vi "UHR-Fleezers Control (host) - 11.0.vi"() -> ()   [LabVIEW 2011] (continued)
            n1358 = Multiply(x=3276.7, y=w1898) -> (x*y=w1899:cluster{"Set 1":dbl, "Set 2":dbl})
            n1359 = To Word Integer(number=w1899) -> (16bit integer=w1911:cluster{"Set 1":i16, "Set 2":i16})
          }
        }
        n1360 = Unbundle By Name(w1883) -> ("Set 1"=w1882:i16, "Set 2"=w1881:i16)
        n1361 = xnode "Read/Write Control"("FPGA VI Reference In"=w1879, "error in"=w1878, "FB Setpoint Set 1"=w1882, "FB Setpoint Set 2"=w1881) -> ("error out"=w1877:errorcluster)  [unwired: 1 out]
      }
      event "Invert GI": Value Change {
        n1362 = event-data() -> ()  [unwired: 7 out]
        n1363 = xnode "Read/Write Control"("FPGA VI Reference In"=w1916, "error in"=w1914, "Invert GI"="Invert GI", "Invert GI 2"="Invert GI") -> ("error out"=w1915:errorcluster)  [unwired: 1 out]
      }
      event "Green FB Setpoint (mV)", "Green FB Gains", "Green FB On/Off", "Current When FB OFF (%)", "Green int current ON count adj": Value Change {
        n1364 = event-data() -> ()  [unwired: 7 out]
        n1365 = local read "Green FB Setpoint (mV)"() -> (w1923:dbl)
        n1366 = local read "Current When FB OFF (%)"() -> (w1926:dbl)
        n1367 = Multiply(x=w1923, y=3.2767) -> (x*y=w1922:dbl)
        n1368 = Multiply(x=w1926, y=655.35) -> (x*y=w1927:dbl)
        n1369 = To Unsigned Word Integer(number=w1927) -> (unsigned 16bit integer=w1925:u16)
        n1370 = local read "Green int current ON count adj"() -> (w1930:u32)
        n1371 = local read "Green FB Gains"() -> (w1929:T14)
        n1372 = local read "Green Laser ON/Interlacing"() -> (w1920:bool)
        n1373 = local read "Green laser mode"() -> (w1919:enum32{"Laser ON", "Laser OFF", "Interlace"})
        n1374 = local read "Green FB On/Off"() -> (w1931:bool)
        n1375 = Equal?(x=w1919, y=enum32{"Laser ON", "Laser OFF", "Interlace"}."Interlace") -> (x = y?=w1917:bool)
        n1376 = Compound Arithmetic op=AND(w1917, w1931, w1920) -> (w1921:bool)
        n1377 = xnode "Read/Write Control"("FPGA VI Reference In"=w1934, "error in"=w1933, "Green FB Setpoint"=w1922, "Green FB On/Off"=w1921, "Current Out"=w1925, "Green int current ON count adj"=w1930, "Green FB Gains"=w1929) -> ("error out"=w1932:errorcluster)  [unwired: 1 out]
      }
      event "Green laser mode", "Green Laser ON/Interlacing": Value Change {
        n1378 = event-data() -> ()  [unwired: 7 out]
        n1379 = local write "Green Laser ON/OFF"("Green Laser ON/Interlacing") -> ()
        n1380 = case shown="True" "Green Laser ON/Interlacing" {
          tunnel: "Green laser mode" -> [_ w1948]
          tunnel: [enum32{"Laser ON", "Laser OFF", "Interlace"}."Laser OFF" ("Green laser mode") w1948] -> w1937
          tunnel: [FALSE w1944] -> w1936
          frame False {
          }
          frame True {
            n1381 = local read "Green FB On/Off"() -> (w1945:bool)
            n1382 = Equal?(x=w1948, y=enum32{"Laser ON", "Laser OFF", "Interlace"}."Interlace") -> (x = y?=w1946:bool)
            n1383 = And(x=w1946, y=w1945) -> (x .and. y?=w1944:bool)
          }
        }
        n1384 = xnode "Read/Write Control"("FPGA VI Reference In"=w1941, "error in"=w1939, "Operating Mode"=w1937, "Operating Mode 2"=w1937, "Green FB On/Off"=w1936) -> ("error out"=w1940:errorcluster)  [unwired: 1 out]
      }
      event "Green Laser ON/OFF": Value Change {
        n1385 = event-data() -> ()  [unwired: 7 out]
        n1386 = property on="Green Laser ON/Interlacing" class="Bool (strict)"("Val(Sgnl)"="Green Laser ON/OFF") -> ()  [unwired: 2 in, 2 out]
      }
      event "Test ttrig": Value Change {
        n1387 = event-data() -> ()  [unwired: 7 out]
        n1388 = xnode "Read/Write Control"("FPGA VI Reference In"=w1953, "error in"=w1952, "TTrig?"=TRUE) -> ("error out"=w1951:errorcluster)  [unwired: 1 out]
      }
      event "Neg. TTrig FPGA": Value Change {
        n1389 = event-data() -> ()  [unwired: 7 out]
        n1390 = xnode "Read/Write Control"("FPGA VI Reference In"=w1957, "error in"=w1956, "TTrig Negate Pos"="Neg. TTrig FPGA") -> ()  [unwired: 2 out]
      }
      event "- phase (APD 1 Gate)", "+ phase (APD 1 Gate)": Value Change {
        n1391 = event-data() -> ()  [unwired: 7 out]
        n1392 = local read "Phase Adj. (APD 1 Gate)"() -> (w1958:i16)
        n1393 = Negate(x=w1958) -> (-x=w1966:i16)
        n1394 = Select(t=w1966, s="- phase (APD 1 Gate)", f=w1958) -> (s? t:f=w1965:i16)
        n1395 = Or(x="- phase (APD 1 Gate)", y="+ phase (APD 1 Gate)") -> (x .or. y?=w1961:bool)
        n1396 = xnode "Read/Write Control"("FPGA VI Reference In"=w1968, "error in"=w1967, "Phase count adjustment (APD 1 Gate)"=w1965) -> ("FPGA VI Reference Out"=w1963:T19, "error out"=w1964:errorcluster)
        n1397 = xnode "Read/Write Control"("FPGA VI Reference In"=w1963, "error in"=w1964, "+ phase (APD 1 Gate)"=w1961) -> ("error out"=w1962:errorcluster)  [unwired: 1 out]
      }
      event "+ phase (APD 2 Gate)", "- phase (APD 2 Gate)": Value Change {
        n1398 = event-data() -> ()  [unwired: 7 out]
        n1399 = local read "Phase Adj. (APD 2 Gate)"() -> (w1969:i16)
        n1400 = Negate(x=w1969) -> (-x=w1977:i16)
        n1401 = Select(t=w1977, s="- phase (APD 2 Gate)", f=w1969) -> (s? t:f=w1976:i16)
        n1402 = Or(x="- phase (APD 2 Gate)", y="+ phase (APD 2 Gate)") -> (x .or. y?=w1972:bool)
        n1403 = xnode "Read/Write Control"("FPGA VI Reference In"=w1979, "error in"=w1978, "Phase count adjustment (APD 2 Gate)"=w1976) -> ("FPGA VI Reference Out"=w1974:T19, "error out"=w1975:errorcluster)
        n1404 = xnode "Read/Write Control"("FPGA VI Reference In"=w1974, "error in"=w1975, "+ phase (APD 2 Gate)"=w1972) -> ("error out"=w1973:errorcluster)  [unwired: 1 out]
      }
      event "Phase Adj. (APD Acq)", "+ phase (APD Acq)", "- phase (APD Acq)": Value Change {
        n1405 = event-data() -> ()  [unwired: 7 out]
        n1406 = local read "Phase Adj. (APD Acq)"() -> (w1982:i16)
        n1407 = Negate(x=w1982) -> (-x=w1988:i16)
        n1408 = Select(t=w1988, s="+ phase (APD Acq)", f=w1982) -> (s? t:f=w1987:i16)
        n1409 = Or(x="+ phase (APD Acq)", y="- phase (APD Acq)") -> (x .or. y?=w1983:bool)
        n1410 = xnode "Read/Write Control"("FPGA VI Reference In"=w1990, "error in"=w1989, "Phase Count Adjustment (APD Acq)"=w1987) -> ("FPGA VI Reference Out"=w1985:T19, "error out"=w1986:errorcluster)
        n1411 = xnode "Read/Write Control"("FPGA VI Reference In"=w1985, "error in"=w1986, "+ phase (APD Acq)"=w1983) -> ("error out"=w1984:errorcluster)  [unwired: 1 out]
      }
      event "Phase adj. (GI)", "+ phase (GI)", "- phase (GI)": Value Change {
        n1412 = event-data() -> ()  [unwired: 7 out]
        n1413 = Negate(x="Phase adj. (GI)") -> (-x=w1999:i16)
        n1414 = Select(t=w1999, s="+ phase (GI)", f="Phase adj. (GI)") -> (s? t:f=w1998:i16)
        n1415 = Or(x="+ phase (GI)", y="- phase (GI)") -> (x .or. y?=w1994:bool)
        n1416 = xnode "Read/Write Control"("FPGA VI Reference In"=w2001, "error in"=w2000, "Phase count adjustment (GI)"=w1998) -> ("FPGA VI Reference Out"=w1996:T19, "error out"=w1997:errorcluster)
        n1417 = xnode "Read/Write Control"("FPGA VI Reference In"=w1996, "error in"=w1997, "+ phase (GI)"=w1994) -> ("error out"=w1995:errorcluster)  [unwired: 1 out]
      }
      event "Phase adj. (GI) 2", "+ phase (GI) 2", "- phase (GI) 2": Value Change {
        n1418 = event-data() -> ()  [unwired: 7 out]
        n1419 = Negate(x="Phase adj. (GI) 2") -> (-x=w2010:i16)
        n1420 = Select(t=w2010, s="+ phase (GI) 2", f="Phase adj. (GI) 2") -> (s? t:f=w2009:i16)
        n1421 = Or(x="+ phase (GI) 2", y="- phase (GI) 2") -> (x .or. y?=w2005:bool)
        n1422 = xnode "Read/Write Control"("FPGA VI Reference In"=w2012, "error in"=w2011, "Phase count adjustment (GI) 2"=w2009) -> ("FPGA VI Reference Out"=w2007:T19, "error out"=w2008:errorcluster)
        n1423 = xnode "Read/Write Control"("FPGA VI Reference In"=w2007, "error in"=w2008, "+ phase (GI) 2"=w2005) -> ("error out"=w2006:errorcluster)  [unwired: 1 out]
      }
      event "Phase adj. (Green FB)", "- phase (Green FB)", "+ phase (Green FB)": Value Change {
        n1424 = event-data() -> ()  [unwired: 7 out]
        n1425 = Negate(x="Phase adj. (Green FB)") -> (-x=w2021:i16)
        n1426 = Select(t=w2021, s="+ phase (Green FB)", f="Phase adj. (Green FB)") -> (s? t:f=w2020:i16)
        n1427 = Or(x="+ phase (Green FB)", y="- phase (Green FB)") -> (x .or. y?=w2016:bool)
        n1428 = xnode "Read/Write Control"("FPGA VI Reference In"=w2023, "error in"=w2022, "Phase count adjustment (Green FB)"=w2020) -> ("FPGA VI Reference Out"=w2018:T19, "error out"=w2019:errorcluster)
        n1429 = xnode "Read/Write Control"("FPGA VI Reference In"=w2018, "error in"=w2019, "+ phase (Green FB)"=w2016) -> ("error out"=w2017:errorcluster)  [unwired: 1 out]
      }
      event "Invert APD Gate", "APD Gate ON Count", "APD Gate OFF Count", "APD Gate", "APD Integration Time (s)", "APD 1 AO Mult.", "APD 2 AO Mult.", "On one out of X cycles": Value Change {
        n1430 = event-data() -> ()  [unwired: 7 out]
        n1431 = Add(x="GI Frequency, ON count", y="GI Frequency, OFF count") -> (x+y=w2027:u32)
        n1432 = Add(x="APD Gate ON Count", y="APD Gate OFF Count") -> (x+y=w2040:u32)
        n1433 = Multiply(x="On one out of X cycles", y=w2027) -> (x*y=w2024:u32)
        "Green FB Count" <- w2024
        n1434 = Subtract(x=w2024, y="GI Frequency, ON count") -> (x-y=w2025:u32)
        n1435 = Multiply(x=w2040, y="On one out of X cycles") -> (x*y=w2039:u32)
        n1436 = Subtract(x=w2039, y="APD Gate ON Count") -> (x-y=w2038:u32)
        n1437 = local read "DMA Update Period (s)"() -> (w2041:dbl)
        n1438 = Multiply(x="APD Integration Time (s)", y=40000000.0) -> (x*y=w2046:dbl)
        n1439 = Reciprocal(x="APD Integration Time (s)") -> (1/x=→"APD Acq Rate (Hz)":dbl)
        n1440 = To Unsigned Long Integer(number=w2046) -> (unsigned 32bit integer=w2030:u32)
        "APD Int. Count" <- w2030
        n1441 = xnode "Read/Write Control"("FPGA VI Reference In"=w2050, "error in"=w2049, "Invert APD Gate"="Invert APD Gate", "APD Gate ON Count"="APD Gate ON Count", "APD Gate OFF Count"=w2038, "APD Acq Rate Count"=w2030, "APD Gate Operating Mode"="APD Gate", "APD 1 AO scale factor"="APD 1 AO Mult.", "APD 2 AO scale factor"="APD 2 AO Mult.", "Green interlace ON count"="GI Frequency, ON count", "Green interlace OFF count"=w2025, "Green interlace ON count 2"="GI Frequency, ON count", "Green interlace OFF count 2"=w2025, "Green FB Count"=w2024) -> ("error out"=w2048:errorcluster)  [unwired: 1 out]
        n1442 = Divide(x=w2041, y="APD Integration Time (s)") -> (x/y=w2044:dbl)
        n1443 = Multiply(x=2.0, y=w2044) -> (x*y=w2043:dbl)
        n1444 = local write "APD Samples/FIFO Acq."(w2044) -> ()
        n1445 = local write "APD Elements/DMA read"(w2043) -> ()
      }
      event "Number of F/B Scans (AOD)", "Scan Speed (nm/s)", "Scan BD", "Initial delta (MHz)", "Step Size (nm)", "Scan Range (nm)": Value Change {
        w2112 = 123.0  # AOM cal (nm/MHz)
        n1446 = event-data() -> ()  [unwired: 7 out]
        n1447 = local read "BD 1 Frequency 1 (MHz)"() -> (w2095:dbl)
        n1448 = local read "AOM X Cal (nm/MHz)"() -> (w2087:dbl)
        n1449 = local read "X RF Frequency Limits (MHz)"() -> (w2099:T16)
        n1450 = local read "Y RF Frequency Limits (MHz)"() -> (w2096:T16)
        n1451 = local read "BD 2 Frequency 1 (MHz)"() -> (w2101:dbl)
        n1452 = Negate(x="Scan Range (nm)") -> (-x=w2065:dbl)
        n1453 = Divide(x=w2065, y=w2087) -> (x/y=w2069:dbl)
        n1454 = Select(t=w2099, s="Scan BD", f=w2096) -> (s? t:f=w2098:T16)
        n1455 = Select(t=w2095, s="Scan BD", f=w2101) -> (s? t:f=w2100:dbl)
        n1456 = Unbundle By Name(w2098) -> ("Maximum"=w2107:dbl, "Minimum"=w2106:dbl)
        n1457 = Add(x=w2069, y=w2100) -> (x+y=w2104:dbl)
        n1458 = Divide(x=w2065, y="Step Size (nm)") -> (x/y=w2084:dbl)
        n1459 = Divide(x="Step Size (nm)", y=w2087) -> (x/y=w2093:dbl)
        n1460 = Absolute Value(x=w2084) -> (abs(x)=w2068:dbl)
        n1461 = Sign(1:w2065) -> (0:w2066:dbl)
        n1462 = In Range and Coerce(upper limit=w2107, x=w2104, lower limit=w2106) -> (coerced(x)=w2103:dbl, In Range?=w2105:bool)
        n1463 = To Unsigned Quad Integer(1:w2068) -> (0:w2083:u64)
        "Scan steps (AOD)" <- w2083
        n1464 = call "IR AOM freq to word.vi"("Frequency In (MHz)"=w2093) -> ("Frequency Word Out (double)"=w2090:dbl)
        n1465 = Multiply(x=w2066, y=w2090) -> (x*y=w2067:dbl)
        n1466 = Subtract(x=w2104, y=w2103) -> (x-y=w2102:dbl)
        n1467 = To Quad Integer(1:w2067) -> (0:w2089:i64)
        "Incr. int (AOD)" <- w2089
        n1468 = Subtract(x=w2069, y=w2102) -> (x-y=w2088:dbl)
        "Scan Range (MHz)" <- w2088
        n1469 = Select(t=w2069, s=w2105, f=w2088) -> (s? t:f=w2108:dbl)
        n1470 = Multiply(x=w2088, y=w2087) -> (x*y=w2086:dbl)
        n1471 = Decrement(x=w2083) -> (x-1=w2136:u64)
        n1472 = Negate(x=w2086) -> (-x=w2082:dbl)
        n1473 = local write "Scan Range (nm)"(w2082) -> ()
        n1474 = Divide(x=w2108, y=w2136) -> (x/y=w2092:dbl)
        "Scan Increment (MHz)" <- w2092
        n1475 = call "IR AOM freq to word.vi"("Frequency In (MHz)"=w2092) -> ("Frequency Word Out (double)"=w2091:dbl)
        n1476 = Divide(x="Step Size (nm)", y="Scan Speed (nm/s)") -> (x/y=w2079:dbl)
        n1477 = To Quad Integer(1:w2091) -> ()  [unwired: 1 out]
        n1478 = local read "Number Interlace Sets"() -> (w2063:u8)
        n1479 = local read "AI Count (ticks)"() -> (w2064:u32)
        n1480 = local read "Total Counts (ticks)"() -> (w2062:u32)
        n1481 = local read "# Samples/trap"() -> (w2094:u32)
        n1482 = Multiply(x=w2064, y=w2063) -> (x*y=w2061:u32)
        n1483 = Divide(x=w2062, y=w2061) -> (x/y=w2060:dbl)
        n1484 = Select(t=w2095, s="Scan BD", f=w2101) -> (s? t:f=w2133:dbl)
        "Initial freq. (MHz)" <- w2133
        n1485 = Add(x=w2108, y=w2133) -> (x+y=→"Final freq. (MHz)":dbl)
        n1486 = Divide(x=w2062, y=40000000.0) -> (x/y=w2078:dbl)
        n1487 = Divide(x=w2079, y=w2078) -> (x/y=w2077:dbl)
        n1488 = To Unsigned Quad Integer(1:w2077) -> (0:w2052:u64)
        n1489 = Quotient & Remainder(x=w2052, y=u64 2) -> (x-y*floor(x/y)=w2056:u64)  [unwired: 1 out]
        n1490 = Equal?(x=w2056, y=u64 0) -> (x = y?=w2054:bool)
        n1491 = Decrement(x=w2052) -> (x-1=w2053:u64)
        n1492 = Select(t=w2052, s=w2054, f=w2053) -> (s? t:f=w2051:u64)
        "Cycles/step (AOD)" <- w2051
        n1493 = xnode "Read/Write Control"("FPGA VI Reference In"=w2144, "error in"=w2143, "Scan steps"=w2083, "Number of scans"="Number of F/B Scans (AOD)", "Cycles per step"=w2051, "Scan freq.  increment"=w2089, "Scan BD"="Scan BD") -> ("error out"=w2142:errorcluster)  [unwired: 1 out]
        n1494 = Multiply(x=w2083, y=w2051) -> (x*y=w2137:u64)
        n1495 = Multiply(x=w2137, y=u64 2) -> (x*y=w2059:u64)
        n1496 = Multiply(x=w2060, y=w2059) -> (x*y=w2058:dbl)
        "Data points/scan (f/b)" <- w2058
        n1497 = Multiply(x=w2058, y="Number of F/B Scans (AOD)") -> (x*y=w2140:dbl)
        "Data points/scans" <- w2140
        n1498 = Divide(x=w2140, y=w2094) -> (x/y=→"N sets should be saved":dbl)
        n1499 = Multiply(x=w2137, y=w2078) -> (x*y=w2076:dbl)
        "Time/Scan (s) (AOD)" <- w2076
        n1500 = Select(t=w2108, s="Scan BD", f=0.0) -> (s? t:f=w2134:dbl)
        n1501 = Select(t=0.0, s="Scan BD", f=w2108) -> (s? t:f=w2130:dbl)
        n1502 = local read "BD 2 Frequency 2 (MHz)"() -> (w2126:dbl)
        n1503 = local read "BD 1 Frequency 2 (MHz)"() -> (w2129:dbl)
        n1504 = Add(x=w2130, y=w2101) -> (x+y=w2127:dbl)
        n1505 = Add(x=w2095, y=w2134) -> (x+y=w2128:dbl)
        n1506 = Multiply(x=w2076, y=2.0) -> (x*y=w2075:dbl)
        n1507 = Multiply(x=w2075, y="Number of F/B Scans (AOD)") -> (x*y=w2072:dbl)
        n1508 = Divide(x=w2072, y=60.0) -> (x/y=→"Time to Finish All (min)":dbl)
        n1509 = Add(x="Trap 2 Bead Size (nm)", y="Trap 1 Bead Size (nm)") -> (x+y=w2116:dbl)
        n1510 = Divide(x=w2116, y=2.0) -> (x/y=w2110:dbl)
        n1511 = local read "Initial delta (MHz)"() -> (w2113:dbl)
        n1512 = Subtract(x=w2127, y=w2126) -> (x-y=w2124:dbl)
        n1513 = Subtract(x=w2128, y=w2129) -> (x-y=w2125:dbl)
        n1514 = Square(x=w2124) -> (x^2=w2123:dbl)
        n1515 = Square(x=w2125) -> (x^2=w2122:dbl)
        n1516 = Add(x=w2122, y=w2123) -> (x+y=w2121:dbl)
        n1517 = Square Root(x=w2121) -> (sqrt(x)=w2120:dbl)
        "Final delta (MHz)" <- w2120
        n1518 = Multiply(x=w2112, y=w2120) -> (x*y=w2119:dbl)
        n1519 = Multiply(x=w2113, y=w2112) -> (x*y=w2111:dbl)
        n1520 = Subtract(x=w2111, y=w2110) -> (x-y=→"Initial sep (nm)":dbl)
        n1521 = Subtract(x=w2119, y=w2110) -> (x-y=→"Final sep (nm)":dbl)
      }
      event "Freq or Amp switch first", "Swap F1 and F2", "Freq switch delay", "Amp switch delay": Value Change {
        n1522 = event-data() -> ()  [unwired: 7 out]
        n1523 = local read "Freq or Amp switch first"() -> (w2145:bool)
        n1524 = local read "Amp switch delay"() -> (w2146:u16)
        n1525 = local read "Freq switch delay"() -> (w2148:u16)
        n1526 = local read "Swap F1 and F2"() -> (w2147:bool)
        n1527 = xnode "Read/Write Control"("FPGA VI Reference In"=w2151, "error in"=w2150, "Freq switch delay"=w2148, "Swap F1 and F2"=w2147, "Amp switch delay"=w2146, "Freq or Amp switch first"=w2145) -> ("error out"=w2149:errorcluster)  [unwired: 1 out]
      }
      event "Scan steps (MCL)", "Number of scans (MCL)", "Scan Range (V)\n(of steps)", "2D or 1D Scan", "N APD Samp/step", "Fast Scan Dir", "Continuous MCL Scanning", "Scan lines (y)": Value Change {
        w2153 = 32767.0 ("y")
        n1528 = event-data() -> ()  [unwired: 7 out]
        n1529 = Select(t="Scan lines (y)", s="2D or 1D Scan", f="Number of scans (MCL)") -> (s? t:f=w2158:u64)
        n1530 = Decrement(x="Scan steps (MCL)") -> (x-1=w2174:u64)
        n1531 = Divide(x="Scan Range (V)\n(of steps)", y=w2174) -> (x/y=w2173:dbl)
        "Desired Scan Incr (V)" <- w2173
        n1532 = local read "APD Integration Time (s)"() -> (w2166:dbl)
        n1533 = Multiply(x=w2173, y=w2153) -> (x*y=w2182:dbl)
        n1534 = Divide(x=w2182, y=10.0) -> (x/y=w2172:dbl)
        "Desired incr (int)" <- w2172
        n1535 = local read "Update Count (MCL)"() -> (w2178:u32)
        n1536 = Round Toward -Infinity(1:w2172) -> (0:w2181:dbl)
        n1537 = To Word Integer(number=w2181) -> (16bit integer=w2156:i16)
        "Actual Incr. int (MCL)" <- w2156
        n1538 = Multiply(x=w2166, y=40000000.0) -> (x*y=w2179:dbl)
        n1539 = Divide(x=w2179, y=w2178) -> (x/y=w2177:dbl)
        n1540 = Multiply(x=i16 10, y=w2156) -> (x*y=w2154:i16)
        n1541 = Multiply(x="N APD Samp/step", y=w2177) -> (x*y=w2176:dbl)
        "Cycles/step (MCL)" <- w2176
        n1542 = Divide(x=w2154, y=w2153) -> (x/y=→"Actual MCL Inc (V)":dbl)
        n1543 = Multiply(x="N APD Samp/step", y="Scan steps (MCL)") -> (x*y=w2168:dbl)
        n1544 = local read "APD Samples/FIFO Acq."() -> (w2165:dbl)
        n1545 = Multiply(x=w2168, y=u64 2) -> (x*y=w2167:dbl)
        "Data points/scan (f+b)" <- w2167
        n1546 = Multiply(x=w2167, y=w2158) -> (x*y=w2185:dbl)
        "Data points/scans (MCL)" <- w2185
        n1547 = Multiply(x=w2166, y=w2167) -> (x*y=w2159:dbl)
        "Time/f+b scan (s) (MCL)" <- w2159
        n1548 = Divide(x=w2185, y=w2165) -> (x/y=→"N sets should be saved (MCL)":dbl)
        n1549 = Multiply(x=w2159, y=w2158) -> (x*y=→"Total Time (s)":dbl)
        n1550 = Not(x="Fast Scan Dir") -> (.not. x?=w2163:bool)
        n1551 = xnode "Read/Write Control"("FPGA VI Reference In"=w2189, "error in"=w2188, "Scan steps (MCL)"="Scan steps (MCL)", "Number of scans (MCL)"=w2158, "Cycles per step (MCL)"=w2176, "Scan freq.  increment (MCL)"=w2156, "1D or 2D Scan?"="2D or 1D Scan", "MCL Scan Axis"=w2163, "Cont. Scan (MCL)"="Continuous MCL Scanning") -> ("error out"=w2187:errorcluster)  [unwired: 1 out]
      }
      event "Read Cal": Value Change {
        w2191 = 1000.0 ("y")
        n1552 = event-data() -> ()  [unwired: 7 out]
        n1553 = local read "Save file name"() -> (w2216:path)
        n1554 = local write "Read Cal"(FALSE ("Read Cal")) -> ()
        n1555 = Strip Path(path=w2216) -> (stripped path=w2215:path)  [unwired: 1 out]
        n1556 = Path To String(path=w2215) -> (string=w2214:string)
        n1557 = Concatenate Strings(w2214, "\\current.cal" ("string")) -> (w2212:string)
        n1558 = String To Path(string=w2212) -> (path=w2211:path)
        n1559 = Open/Create/Replace File(file path (use dialog)=w2211, operation (0:open)=T25."open", access (0:read/write)=enum16{"read/write", "read-only", "write-only"}."read-only") -> (refnum out=w2219:refnum<file>, error out=w2205:errorcluster)  [unwired: 1 in, 3 out]
        n1560 = Deny Access(4:w2205, 7:w2219) -> (0:w2204:errorcluster, 3:w2210:refnum<file>)  [unwired: 1 out]
        n1561 = Read from Binary File(5:0.0, 8:w2204, 9:T24."big-endian, network order" ("byte order (0:big-endian, network order)"), 10:-1 ("count (1)"), 11:w2210) -> (0:w2203:errorcluster, 2:w2201:dbl[], 3:w2206:refnum<file>)  [unwired: 2 out]
        n1562 = Array To Cluster(array=w2201) -> (cluster=w2200:T27)
        n1563 = Unbundle(w2200) -> ("[0]"=w2199:dbl, "[1]"=w2198:dbl, "[2]"=w2197:dbl, "[3]"=w2196:dbl, "[4]"=w2195:dbl, "[5]"=w2194:dbl)
        n1564 = Close File(refnum=w2206, error in=w2203) -> (error out=→"Read cal error":errorcluster)  [unwired: 1 out]
        n1565 = Multiply(x=w2194, y=w2191) -> (x*y=w2192:dbl)
        n1566 = local write "T2 kappa_x (pN/nm)"(w2196) -> ()
        n1567 = local write "T1 kappa_x (pN/nm)"(w2197) -> ()
        n1568 = local write "T1 alpha_x (nm/V)"(w2199) -> ()
        n1569 = local write "T2 alpha_x (nm/V)"(w2198) -> ()
        n1570 = Multiply(x=w2195, y=w2191) -> (x*y=w2193:dbl)
        n1571 = local write "T1 offset_x (mV)"(w2193) -> ()
        n1572 = local write "T2 offset_x (mV)"(w2192) -> ()
      }
      event "Abort MCL Scan": Value Change {
        n1573 = event-data() -> ()  [unwired: 7 out]
        n1574 = local write "MCL Scanning"(FALSE ("MCL Scanning")) -> ()
        n1575 = xnode "Read/Write Control"("FPGA VI Reference In"=w2224, "error in"=w2223, "Abort scan (MCL)"="Abort MCL Scan") -> ("error out"=w2222:errorcluster)  [unwired: 1 out]
      }
      event "Update Count (MCL)": Value Change {
        n1576 = event-data() -> ()  [unwired: 7 out]
        n1577 = xnode "Read/Write Control"("FPGA VI Reference In"=w2228, "error in"=w2227, "MCL count"="Update Count (MCL)") -> ("error out"=w2226:errorcluster)  [unwired: 1 out]
      }
      event "Phase adjust (MCL)", "+ phase (MCL)", "- phase (MCL)": Value Change {
        n1578 = event-data() -> ()  [unwired: 7 out]
        n1579 = Negate(x="Phase adjust (MCL)") -> (-x=w2237:i16)
        n1580 = Select(t=w2237, s="- phase (MCL)", f="Phase adjust (MCL)") -> (s? t:f=w2235:i16)
        n1581 = Or(x="- phase (MCL)", y="+ phase (MCL)") -> (x .or. y?=w2230:bool)
        n1582 = xnode "Read/Write Control"("FPGA VI Reference In"=w2239, "error in"=w2238, "Phase count adjustment (MCL)"=w2235) -> ("FPGA VI Reference Out"=w2231:T19, "error out"=w2232:errorcluster)
        n1583 = xnode "Read/Write Control"("FPGA VI Reference In"=w2231, "error in"=w2232, "+ phase (MCL)"=w2230) -> ("error out"=w2229:errorcluster)  [unwired: 1 out]
      }
      event "Abort AOD Scan": Value Change {
        n1584 = event-data() -> ()  [unwired: 7 out]
        n1585 = xnode "Read/Write Control"("FPGA VI Reference In"=w2243, "error in"=w2242, "Abort scan"="Abort AOD Scan") -> ("error out"=w2241:errorcluster)  [unwired: 1 out]
      }
      event "Continuous AOD Scanning": Value Change {
        n1586 = event-data() -> ()  [unwired: 7 out]
        n1587 = xnode "Read/Write Control"("FPGA VI Reference In"=w2247, "error in"=w2246, "Cont. Scan"="Continuous AOD Scanning") -> ("error out"=w2245:errorcluster)  [unwired: 1 out]
      }
      event "Index": Value Change {
        n1588 = event-data() -> ()  [unwired: 7 out]
        n1589 = call "Create new save file.vi"("Insert"="", "Ext"=".dat" ("string"), "Index In"="Index") -> ("Path Out"=→"Save file name":path, "Index Out"=w2248:dbl)
        "Save index" <- w2248
        n1590 = local write "Index"(w2248) -> ()
      }
      event "AO1", "AO2": Value Change {
        w2263 = 10.0 ("y")
        w2262 = 32767.0 ("y")
        n1591 = event-data() -> ()  [unwired: 7 out]
        n1592 = local read "AO2"() -> (w2261:dbl)
        n1593 = local read "AO1"() -> (w2258:dbl)
        n1594 = Multiply(x=w2258, y=w2262) -> (x*y=w2257:dbl)
        n1595 = Multiply(x=w2261, y=w2262) -> (x*y=w2260:dbl)
        n1596 = Divide(x=w2257, y=w2263) -> (x/y=w2256:dbl)
        n1597 = Divide(x=w2260, y=w2263) -> (x/y=w2259:dbl)
        n1598 = To Word Integer(number=w2256) -> (16bit integer=w2264:i16)
        n1599 = To Word Integer(number=w2259) -> (16bit integer=w2265:i16)
        n1600 = xnode "Read/Write Control"("FPGA VI Reference In"=w2255, "error in"=w2254, "AO1"=w2264, "AO2"=w2265) -> ("error out"=w2253:errorcluster)  [unwired: 1 out]
      }
      event "Inject Pump 1": Value Change {
        n1601 = event-data() -> ()  [unwired: 7 out]
        n1602 = local read "Use Harvard pumps\nfor beads (else Chemyx)"() -> (w2267:bool)
        n1603 = case shown="True" w2267 {
          tunnel: "Inject Pump 1" -> [w2271 w2309]
          tunnel: w2266 -> [_ w2310]
          frame False {
            n1604 = local read "Pump write delay (ms)"() -> (w2270:dbl)
            n1605 = local read "Chemyx Syringe Pump Serial Port"() -> (w2269:refnum<visa-resource-name>)
            n1606 = case shown="True" w2271 {
              tunnel: w2270 -> [w2277 w2291]
              tunnel: w2269 -> [w2274 w2290]
              frame False {
                n1607 = flat-sequence {
                  tunnel: w2274 -> [w2278]
                  tunnel: [w2278] -> w2275
                  tunnel: w2277 -> [_]
                  tunnel: [w2281] -> w2276
                  tunnel: w2275 -> [w2281]
                  tunnel: w2276 -> [w2282]
                  tunnel: [w2282] -> w2272
                  tunnel: [w2284] -> w2273
                  tunnel: w2272 -> [w2284]
                  tunnel: w2273 -> [w2286]
                  frame #0 {
                    n1608 = call "Write to pump.vi"("string"="enter pump1", "VISA resource name"=w2278) -> ()  [unwired: 1 out]
                  }
                  frame #1 {
                    n1609 = Wait (ms)(milliseconds to wait="Pump pause delay (ms)") -> ()  [unwired: 1 out]
                  }
                  frame #2 {
                    n1610 = call "Write to pump.vi"("string"="stop", "VISA resource name"=w2282) -> ()  [unwired: 1 out]
                  }
                  frame #3 {
                    n1611 = Wait (ms)(milliseconds to wait=u32 500) -> ()  [unwired: 1 out]
                  }
                  frame #4 {
                    n1612 = call "Write to pump.vi"("string"="stop", "VISA resource name"=w2286) -> ()  [unwired: 1 out]
                  }
                }
              }
              frame True {
                n1613 = flat-sequence {
                  tunnel: w2290 -> [w2300]
                  tunnel: w2291 -> [w2295]
                  tunnel: w2291 -> [w2302]
                  tunnel: w2290 -> [w2303]
                  tunnel: [w2303] -> w2288
                  tunnel: [w2305] -> w2289
                  tunnel: w2288 -> [w2305]
                  tunnel: w2289 -> [w2307]
                  frame #0 {
                    n1614 = local read "All Pump Parameters"() -> (w2294:T5)
                    n1615 = Unbundle By Name(w2294) -> ("Pump 1"=w2301:T28)
                    n1616 = call "Set pump parameters.vi"("Pump write delay (ms)"=w2295, "Volume (uL)"="Ch 1 Inject Volume (uL)", "Rate (uL/h)"="Ch 1 Inject Rate (ul/h)", "Units"=4.0, "Pump #"=1.0, "Pump Parameters In"=w2301, "VISA resource name"=w2300) -> ("Pump Parameters Out"=w2293:T28)  [unwired: 3 in]
                    n1617 = Bundle By Name(cluster=w2294, "Pump 1"=w2293) -> (w2292:T5)
                    n1618 = local write "All Pump Parameters"(w2292) -> ()
                  }
                  frame #1 {
                    n1619 = Wait (ms)(milliseconds to wait=w2302) -> ()  [unwired: 1 out]
                  }
                  frame #2 {
                    n1620 = call "Write to pump.vi"("string"="start", "VISA resource name"=w2303) -> ()  [unwired: 1 out]
                  }
                  frame #3 {
                    n1621 = Wait (ms)(milliseconds to wait=u32 500) -> ()  [unwired: 1 out]
                  }
                  frame #4 {
                    n1622 = call "Write to pump.vi"("string"="start", "VISA resource name"=w2307) -> ()  [unwired: 1 out]
                  }
                }
              }
            }
          }
          frame True {
            n1623 = case shown="False" w2309 {
              tunnel: w2310 -> [w2311 w2321]
              frame False {
                n1624 = flat-sequence {
                  tunnel: w2311 -> [w2313]
                  frame #0 {
                    n1625 = local write "Flushing P1"(FALSE ("Flushing P1")) -> ()
                    n1626 = Concatenate Strings("stop" ("string"), "\r") -> (w2315:string)
                    n1627 = VISA Write(VISA resource name=w2313, write buffer=w2315) -> ()  [unwired: 1 in, 3 out]
                  }
                  frame #1 {
                    n1628 = property on="Clear Volume P1" class="Bool (strict)"("Val(Sgnl)"=TRUE ("Value (Signaling)")) -> ()  [unwired: 2 in, 2 out]
                  }
                }
              }
              frame True {
                n1629 = local read "Normal Flow Rate (ul/h) P1"() -> (w2319:dbl)
                n1630 = Number To Decimal String(number=w2319) -> (decimal integer string=w2325:string)  [unwired: 1 in]
                n1631 = Concatenate Strings("irate  " ("string"), w2325, " u/h" ("string"), "\r") -> (w2323:string)
                n1632 = VISA Write(VISA resource name=w2321, write buffer=w2323) -> (VISA resource name out=w2320:refnum<visa-resource-name>)  [unwired: 1 in, 2 out]
                n1633 = Concatenate Strings("irun" ("string"), "\r") -> (w2327:string)
                n1634 = VISA Write(VISA resource name=w2320, write buffer=w2327) -> ()  [unwired: 1 in, 3 out]
              }
            }
          }
        }
      }
      event "Inject Pump 3": Value Change {
        n1635 = event-data() -> ()  [unwired: 7 out]
        n1636 = local read "Use Harvard pumps\nfor beads (else Chemyx)"() -> (w2330:bool)
        n1637 = case shown="True" w2330 {
          tunnel: "Inject Pump 3" -> [w2334 w2373]
          tunnel: w2329 -> [_ w2372]
          frame False {
            n1638 = local read "Pump write delay (ms)"() -> (w2333:dbl)
            n1639 = case shown="True" w2334 {
              tunnel: w2333 -> [w2340 w2354]
              tunnel: "Chemyx Syringe Pump Serial Port" -> [w2337 w2353]
              frame False {
                n1640 = flat-sequence {
                  tunnel: w2337 -> [w2341]
                  tunnel: [w2341] -> w2338
                  tunnel: w2340 -> [_]
                  tunnel: [w2344] -> w2339
                  tunnel: w2338 -> [w2344]
                  tunnel: w2339 -> [w2345]
                  tunnel: [w2345] -> w2335
                  tunnel: [w2347] -> w2336
                  tunnel: w2335 -> [w2347]
                  tunnel: w2336 -> [w2349]
                  frame #0 {
                    n1641 = call "Write to pump.vi"("string"="enter pump3", "VISA resource name"=w2341) -> ()  [unwired: 1 out]
                  }
                  frame #1 {
                    n1642 = local read "Pump pause delay (ms)"() -> (w2343:u32)
                    n1643 = Wait (ms)(milliseconds to wait=w2343) -> ()  [unwired: 1 out]
                  }
                  frame #2 {
                    n1644 = call "Write to pump.vi"("string"="stop", "VISA resource name"=w2345) -> ()  [unwired: 1 out]
                  }
                  frame #3 {
                    n1645 = Wait (ms)(milliseconds to wait=u32 0) -> ()  [unwired: 1 out]
                  }
                  frame #4 {
                    n1646 = call "Write to pump.vi"("string"="stop", "VISA resource name"=w2349) -> ()  [unwired: 1 out]
                  }
                }
              }
              frame True {
                n1647 = flat-sequence {
                  tunnel: w2353 -> [w2363]
                  tunnel: w2354 -> [w2358]
                  tunnel: w2354 -> [w2365]
                  tunnel: w2353 -> [w2366]
                  tunnel: [w2366] -> w2352
                  tunnel: [w2369] -> w2351
                  tunnel: w2352 -> [w2369]
                  tunnel: w2351 -> [w2370]
                  frame #0 {
                    n1648 = local read "All Pump Parameters"() -> (w2357:T5)
                    n1649 = Unbundle By Name(w2357) -> ("Pump 3"=w2364:T28)
                    n1650 = call "Set pump parameters.vi"("Pump write delay (ms)"=w2358, "Volume (uL)"="Ch 3 Inject Volume (uL)", "Rate (uL/h)"="Ch 3 Inject Rate (ul/h)", "Units"=4.0, "Pump #"=3.0, "Pump Parameters In"=w2364, "VISA resource name"=w2363) -> ("Pump Parameters Out"=w2356:T28)  [unwired: 3 in]
                    n1651 = Bundle By Name(cluster=w2357, "Pump 3"=w2356) -> (w2355:T5)
                    n1652 = local write "All Pump Parameters"(w2355) -> ()
                  }
                  frame #1 {
                    n1653 = Wait (ms)(milliseconds to wait=w2365) -> ()  [unwired: 1 out]
                  }
                  frame #2 {
                    n1654 = call "Write to pump.vi"("string"="start", "VISA resource name"=w2366) -> ()  [unwired: 1 out]
                  }
                  frame #3 {
                    n1655 = Wait (ms)(milliseconds to wait=u32 500) -> ()  [unwired: 1 out]
                  }
                  frame #4 {
                    n1656 = call "Write to pump.vi"("string"="start", "VISA resource name"=w2370) -> ()  [unwired: 1 out]
                  }
                }
              }
            }
          }
          frame True {
            n1657 = case shown="False" w2373 {
              tunnel: w2372 -> [w2374 w2381]
              frame False {
                n1658 = flat-sequence {
                  tunnel: w2374 -> [w2376]
                  frame #0 {
                    n1659 = local write "Flushing P3"(FALSE ("Flushing P3")) -> ()
                    n1660 = Concatenate Strings("stop" ("string"), "\r") -> (w2378:string)
                    n1661 = VISA Write(VISA resource name=w2376, write buffer=w2378) -> ()  [unwired: 1 in, 3 out]
                  }
                  frame #1 {
                    n1662 = property on="Clear Volume P3" class="Bool (strict)"("Val(Sgnl)"=TRUE ("Value (Signaling)")) -> ()  [unwired: 2 in, 2 out]
                  }
                }
              }
              frame True {
                n1663 = local read "Normal Flow Rate (ul/h) P3"() -> (w2382:dbl)
                n1664 = Number To Decimal String(number=w2382) -> (decimal integer string=w2388:string)  [unwired: 1 in]
                n1665 = Concatenate Strings("irate  " ("string"), w2388, " u/h" ("string"), "\r") -> (w2386:string)
                n1666 = VISA Write(VISA resource name=w2381, write buffer=w2386) -> (VISA resource name out=w2384:refnum<visa-resource-name>)  [unwired: 1 in, 2 out]
                n1667 = Concatenate Strings("irun" ("string"), "\r") -> (w2390:string)
                n1668 = VISA Write(VISA resource name=w2384, write buffer=w2390) -> ()  [unwired: 1 in, 3 out]
              }
            }
          }
        }
      }
      event "Inject Pump 2": Value Change {
        n1669 = event-data() -> ()  [unwired: 7 out]
        n1670 = local read "Pump write delay (ms)"() -> (w2394:dbl)
        n1671 = flat-sequence {
          tunnel: w2392 -> [w2407]
          tunnel: w2394 -> [w2403]
          tunnel: "Inject Pump 2" -> [_]
          tunnel: w2394 -> [w2409]
          tunnel: w2392 -> [w2410]
          frame #0 {
            n1672 = local read "All Pump Parameters"() -> (w2402:T5)
            n1673 = Multiply(x=60.0, y="Flush Center Ch Rate (ul/m)") -> (x*y=w2399:dbl)
            n1674 = Unbundle By Name(w2402) -> ("Pump 2"=w2408:T28)
            n1675 = call "Set pump parameters.vi"("Pump write delay (ms)"=w2403, "Volume (uL)"="Flush Center Ch Volume (uL)", "Rate (uL/h)"=w2399, "Units"=3.0, "Pump #"=2.0, "Pump Parameters In"=w2408, "VISA resource name"=w2407) -> ("Pump Parameters Out"=w2401:T28)  [unwired: 3 in]
            n1676 = Bundle By Name(cluster=w2402, "Pump 2"=w2401) -> (w2400:T5)
            n1677 = local write "All Pump Parameters"(w2400) -> ()
            n1678 = Add(x="Flush Center Ch Volume (uL)", y="Total Volume\nFlushed (uL)") -> (x+y=w2396:dbl)
            n1679 = local write "Total Volume\nFlushed (uL)"(w2396) -> ()
          }
          frame #1 {
            n1680 = Wait (ms)(milliseconds to wait=w2409) -> ()  [unwired: 1 out]
          }
          frame #2 {
            n1681 = call "Write to pump.vi"("string"="start", "VISA resource name"=w2410) -> ()  [unwired: 1 out]
          }
        }
        n1682 = local read "Chemyx Syringe Pump Serial Port"() -> (w2392:refnum<visa-resource-name>)
      }
      event "Sample Channel\nFlow": Value Change {
        n1683 = event-data() -> ()  [unwired: 7 out]
        n1684 = Select(t="irun" ("string"), s="Sample Channel\nFlow", f="stop" ("string")) -> (s? t:f=w2414:string)
        n1685 = Concatenate Strings(w2414, "\r") -> (w2417:string)
        n1686 = VISA Write(VISA resource name=w2412, write buffer=w2417) -> ()  [unwired: 1 in, 3 out]
      }
      event "Start Flow": Value Change {
        n1687 = event-data() -> ()  [unwired: 7 out]
        n1688 = local write "Sample Channel\nFlow"(TRUE ("Sample Channel\nFlow")) -> ()
        n1689 = local write "Start Flow"(FALSE ("Start Flow")) -> ()
        n1690 = Concatenate Strings("irun" ("string"), "\r") -> (w2423:string)
        n1691 = VISA Write(VISA resource name=w2419, write buffer=w2423) -> ()  [unwired: 1 in, 3 out]
      }
      event "Stop Flow": Value Change {
        w2425 = FALSE ("Stop Flow")
        n1692 = event-data() -> ()  [unwired: 7 out]
        n1693 = local write "Stop Flow"(w2425) -> ()
        n1694 = local write "Sample Channel\nFlow"(w2425) -> ()
        n1695 = Concatenate Strings("stop" ("string"), "\r") -> (w2428:string)
        n1696 = VISA Write(VISA resource name=w2426, write buffer=w2428) -> ()  [unwired: 1 in, 3 out]
      }
      event "Flow rate (uL/h)": Value Change {
        n1697 = event-data() -> ()  [unwired: 7 out]
        n1698 = Number To Decimal String(number="Flow rate (uL/h)") -> (decimal integer string=w2435:string)  [unwired: 1 in]
        n1699 = Concatenate Strings("irate  " ("string"), w2435, " u/h" ("string"), "\r") -> (w2434:string)
        n1700 = VISA Write(VISA resource name=w2431, write buffer=w2434) -> ()  [unwired: 1 in, 3 out]
      }
      event "Flush Sample": Value Change {
        n1701 = event-data() -> ()  [unwired: 7 out]
        n1702 = flat-sequence {
          tunnel: w2440 -> [w2468]
          tunnel: [w2448] -> w2439
          tunnel: [w2442] -> w2437
          tunnel: w2439 -> [w2472]
          tunnel: [w2472] -> w2438
          tunnel: w2437 -> [w2471]
          tunnel: w2438 -> [w2477]
          frame #0 {
            # "set paramaters (rate, volume) for flush, clear volume"
            n1703 = Number To Decimal String(number="Flush rate (uL/m)") -> (decimal integer string=w2464:string)  [unwired: 1 in]
            n1704 = Concatenate Strings("irate  " ("string"), w2464, " u/m" ("string"), "\r") -> (w2466:string)
            n1705 = VISA Write(VISA resource name=w2468, write buffer=w2466) -> (VISA resource name out=w2462:refnum<visa-resource-name>)  [unwired: 1 in, 2 out]
            n1706 = Reciprocal(x="Flush rate (uL/m)") -> (1/x=w2445:dbl)
            n1707 = Number To Decimal String(number="Volume (uL)") -> (decimal integer string=w2453:string)  [unwired: 1 in]
            n1708 = Multiply(x="Volume (uL)", y=w2445) -> (x*y=w2444:dbl)
            n1709 = Concatenate Strings("tvolume  " ("string"), w2453, " u" ("string"), "\r") -> (w2451:string)
            n1710 = Multiply(x=w2444, y=60000.0) -> (x*y=w2442:dbl)
            n1711 = VISA Write(VISA resource name=w2462, write buffer=w2451) -> (VISA resource name out=w2450:refnum<visa-resource-name>)  [unwired: 1 in, 2 out]
            n1712 = Concatenate Strings("cvolume" ("string"), "\r") -> (w2449:string)
            n1713 = VISA Write(VISA resource name=w2450, write buffer=w2449) -> (VISA resource name out=w2460:refnum<visa-resource-name>)  [unwired: 1 in, 2 out]
            n1714 = Concatenate Strings("irun" ("string"), "\r") -> (w2458:string)
            n1715 = VISA Write(VISA resource name=w2460, write buffer=w2458) -> (VISA resource name out=w2448:refnum<visa-resource-name>)  [unwired: 1 in, 2 out]
          }
          frame #1 {
            # "Have to wait until\nflow is done to reset\nrate"
            n1716 = Add(x=w2471, y=100.0) -> (x+y=w2470:dbl)
            n1717 = Wait (ms)(milliseconds to wait=w2470) -> ()  [unwired: 1 out]
          }
          frame #2 {
            # "reset flow rate to usual flow rate"
            n1718 = local read "Flow rate (uL/h)"() -> (w2483:dbl)
            n1719 = Number To Decimal String(number=w2483) -> (decimal integer string=w2481:string)  [unwired: 1 in]
            n1720 = Concatenate Strings("irate  " ("string"), w2481, " u/h" ("string"), "\r") -> (w2479:string)
            n1721 = VISA Write(VISA resource name=w2477, write buffer=w2479) -> (VISA resource name out=w2473:refnum<visa-resource-name>)  [unwired: 1 in, 2 out]
            n1722 = Concatenate Strings("cvolume" ("string"), "\r") -> (w2474:string)
            n1723 = VISA Write(VISA resource name=w2473, write buffer=w2474) -> ()  [unwired: 1 in, 3 out]
          }
        }
      }
      event "Flush Pump 3": Value Change {
        n1724 = event-data() -> ()  [unwired: 7 out]
        n1725 = flat-sequence {
          tunnel: w2484 -> [w2487]
          frame #0 {
            # "set paramaters (rate, volume) for flush, clear volume"
            n1726 = Number To Decimal String(number="Flush rate (uL/m) P3") -> (decimal integer string=w2509:string)  [unwired: 1 in]
            n1727 = local write "Inject Pump 3"(TRUE ("Inject Pump 3")) -> ()
            n1728 = Concatenate Strings("irate  " ("string"), w2509, " u/m" ("string"), "\r") -> (w2511:string)
            n1729 = VISA Write(VISA resource name=w2487, write buffer=w2511) -> (VISA resource name out=w2507:refnum<visa-resource-name>)  [unwired: 1 in, 2 out]
            n1730 = Reciprocal(x="Flush rate (uL/m) P3") -> (1/x=w2491:dbl)
            n1731 = Number To Decimal String(number="Volume (uL) P3") -> (decimal integer string=w2498:string)  [unwired: 1 in]
            n1732 = Multiply(x="Volume (uL) P3", y=w2491) -> (x*y=w2490:dbl)
            n1733 = Concatenate Strings("tvolume  " ("string"), w2498, " u" ("string"), "\r") -> (w2496:string)
            n1734 = Multiply(x=w2490, y=60.0) -> (x*y=→"HP3 Flush Time (s)":dbl)
            n1735 = VISA Write(VISA resource name=w2507, write buffer=w2496) -> (VISA resource name out=w2495:refnum<visa-resource-name>)  [unwired: 1 in, 2 out]
            n1736 = Concatenate Strings("cvolume" ("string"), "\r") -> (w2494:string)
            n1737 = VISA Write(VISA resource name=w2495, write buffer=w2494) -> (VISA resource name out=w2505:refnum<visa-resource-name>)  [unwired: 1 in, 2 out]
            n1738 = Concatenate Strings("irun" ("string"), "\r") -> (w2503:string)
            n1739 = VISA Write(VISA resource name=w2505, write buffer=w2503) -> ()  [unwired: 1 in, 3 out]
          }
          frame #1 {
            "Flushing P3" <- TRUE ("Flushing P3")
          }
        }
      }
      event "Flush Pump 1": Value Change {
        n1740 = event-data() -> ()  [unwired: 7 out]
        n1741 = flat-sequence {
          tunnel: [w2525] -> w2515
          tunnel: w2514 -> [w2518]
          tunnel: w2515 -> [_]
          frame #0 {
            # "set paramaters (rate, volume) for flush, clear volume"
            n1742 = local write "Inject Pump 1"(TRUE ("Inject Pump 1")) -> ()
            n1743 = Number To Decimal String(number="Flush rate (uL/m) P1") -> (decimal integer string=w2541:string)  [unwired: 1 in]
            n1744 = Concatenate Strings("irate  " ("string"), w2541, " u/m" ("string"), "\r") -> (w2543:string)
            n1745 = VISA Write(VISA resource name=w2518, write buffer=w2543) -> (VISA resource name out=w2539:refnum<visa-resource-name>)  [unwired: 1 in, 2 out]
            n1746 = Reciprocal(x="Flush rate (uL/m) P1") -> (1/x=w2522:dbl)
            n1747 = Number To Decimal String(number="Volume (uL) P1") -> (decimal integer string=w2530:string)  [unwired: 1 in]
            n1748 = Multiply(x="Volume (uL) P1", y=w2522) -> (x*y=w2521:dbl)
            n1749 = Concatenate Strings("tvolume  " ("string"), w2530, " u" ("string"), "\r") -> (w2528:string)
            n1750 = Multiply(x=w2521, y=60.0) -> (x*y=→"HP1 Flush Time (s)":dbl)
            n1751 = VISA Write(VISA resource name=w2539, write buffer=w2528) -> (VISA resource name out=w2527:refnum<visa-resource-name>)  [unwired: 1 in, 2 out]
            n1752 = Concatenate Strings("cvolume" ("string"), "\r") -> (w2526:string)
            n1753 = VISA Write(VISA resource name=w2527, write buffer=w2526) -> (VISA resource name out=w2537:refnum<visa-resource-name>)  [unwired: 1 in, 2 out]
            n1754 = Concatenate Strings("irun" ("string"), "\r") -> (w2535:string)
            n1755 = VISA Write(VISA resource name=w2537, write buffer=w2535) -> (VISA resource name out=w2525:refnum<visa-resource-name>)  [unwired: 1 in, 2 out]
          }
          frame #1 {
            "Flushing P1" <- TRUE ("Flushing P3")
          }
        }
      }
      event "Clear Volume": Value Change {
        n1756 = event-data() -> ()  [unwired: 7 out]
        n1757 = Concatenate Strings("cvolume" ("string"), "\r") -> (w2547:string)
        n1758 = VISA Write(VISA resource name=w2546, write buffer=w2547) -> ()  [unwired: 1 in, 3 out]
      }
      event "Clear Volume P3": Value Change {
        n1759 = event-data() -> ()  [unwired: 7 out]
        n1760 = Concatenate Strings("cvolume" ("string"), "\r") -> (w2553:string)
        n1761 = VISA Write(VISA resource name=w2552, write buffer=w2553) -> ()  [unwired: 1 in, 3 out]
        n1762 = local write "Clear Volume P3"(FALSE ("Clear Volume P3")) -> ()
      }
      event "Clear Volume P1": Value Change {
        n1763 = event-data() -> ()  [unwired: 7 out]
        n1764 = Concatenate Strings("cvolume" ("string"), "\r") -> (w2558:string)
        n1765 = local write "Clear Volume P1"(FALSE ("Clear Volume P1")) -> ()
        n1766 = VISA Write(VISA resource name=w2557, write buffer=w2558) -> ()  [unwired: 1 in, 3 out]
      }
      event "Display On P3": Value Change {
        n1767 = event-data() -> ()  [unwired: 7 out]
        n1768 = Select(t="dim 100", s="Display On P3", f="dim 0") -> (s? t:f=w2564:string)
        n1769 = Concatenate Strings(w2564, "\r") -> (w2566:string)
        n1770 = VISA Write(VISA resource name=w2561, write buffer=w2566) -> ()  [unwired: 1 in, 3 out]
      }
      event "Display On P1": Value Change {
        n1771 = event-data() -> ()  [unwired: 7 out]
        n1772 = Select(t="dim 100", s="Display On P1", f="dim 0") -> (s? t:f=w2571:string)
        n1773 = Concatenate Strings(w2571, "\r") -> (w2573:string)
        n1774 = VISA Write(VISA resource name=w2568, write buffer=w2573) -> ()  [unwired: 1 in, 3 out]
      }
      event "Retract Pump 3": Value Change {
        n1775 = event-data() -> ()  [unwired: 7 out]
        n1776 = local write "Retract Pump 3"(FALSE ("Retract Pump 3")) -> ()
        n1777 = case shown="True" "Retract Pump 3" {
          tunnel: w2575 -> [_ w2578]
          frame False {
          }
          frame True {
            n1778 = Number To Decimal String(number="Retract Rate (uL/m)") -> (decimal integer string=w2596:string)  [unwired: 1 in]
            n1779 = Concatenate Strings("wrate  " ("string"), w2596, " u/m" ("string"), "\r") -> (w2598:string)
            n1780 = VISA Write(VISA resource name=w2578, write buffer=w2598) -> (VISA resource name out=w2589:refnum<visa-resource-name>)  [unwired: 1 in, 2 out]
            n1781 = Number To Decimal String(number="Retract Vol 3 (uL)") -> (decimal integer string=w2591:string)  [unwired: 1 in]
            n1782 = Concatenate Strings("tvolume  " ("string"), w2591, " u" ("string"), "\r") -> (w2588:string)
            n1783 = VISA Write(VISA resource name=w2589, write buffer=w2588) -> (VISA resource name out=w2584:refnum<visa-resource-name>)  [unwired: 1 in, 2 out]
            n1784 = Concatenate Strings("cvolume" ("string"), "\r") -> (w2585:string)
            n1785 = VISA Write(VISA resource name=w2584, write buffer=w2585) -> (VISA resource name out=w2579:refnum<visa-resource-name>)  [unwired: 1 in, 2 out]
            n1786 = Concatenate Strings("wrun" ("string"), "\r") -> (w2580:string)
            n1787 = VISA Write(VISA resource name=w2579, write buffer=w2580) -> ()  [unwired: 1 in, 3 out]
          }
        }
      }
      event "Retract Pump 1": Value Change {
        n1788 = event-data() -> ()  [unwired: 7 out]
        n1789 = local write "Retract Pump 1"(FALSE ("Retract Pump 1")) -> ()
        n1790 = case shown="True" "Retract Pump 1" {
          tunnel: w2600 -> [_ w2605]
          frame False {
          }
          frame True {
            n1791 = local read "Retract Rate (uL/m)"() -> (w2603:dbl)
            n1792 = Number To Decimal String(number=w2603) -> (decimal integer string=w2621:string)  [unwired: 1 in]
            n1793 = Concatenate Strings("wrate  " ("string"), w2621, " u/m" ("string"), "\r") -> (w2623:string)
            n1794 = VISA Write(VISA resource name=w2605, write buffer=w2623) -> (VISA resource name out=w2615:refnum<visa-resource-name>)  [unwired: 1 in, 2 out]
            n1795 = Number To Decimal String(number="Retract Vol 1 (uL)") -> (decimal integer string=w2617:string)  [unwired: 1 in]
            n1796 = Concatenate Strings("tvolume  " ("string"), w2617, " u" ("string"), "\r") -> (w2614:string)
            n1797 = VISA Write(VISA resource name=w2615, write buffer=w2614) -> (VISA resource name out=w2611:refnum<visa-resource-name>)  [unwired: 1 in, 2 out]
            n1798 = Concatenate Strings("cvolume" ("string"), "\r") -> (w2612:string)
            n1799 = VISA Write(VISA resource name=w2611, write buffer=w2612) -> (VISA resource name out=w2606:refnum<visa-resource-name>)  [unwired: 1 in, 2 out]
            n1800 = Concatenate Strings("wrun" ("string"), "\r") -> (w2607:string)
            n1801 = VISA Write(VISA resource name=w2606, write buffer=w2607) -> ()  [unwired: 1 in, 3 out]
          }
        }
      }
      event "Flip Green Filter": Value Change {
        n1802 = event-data() -> ()  [unwired: 7 out]
        n1803 = Not(x="Flip Green Filter") -> (.not. x?=w2625:bool)
        n1804 = local write "Flip Green Filter"(w2625) -> ()
        n1805 = flat-sequence {
          tunnel: w2633 -> [w2638]
          tunnel: w2632 -> [w2637]
          tunnel: [w2635] -> w2630
          tunnel: [w2634] -> w2629
          tunnel: [w2640] -> w2628
          tunnel: w2630 -> [w2640]
          tunnel: [w2639] -> w2627
          tunnel: w2629 -> [w2639]
          tunnel: w2628 -> [w2644]
          tunnel: w2627 -> [w2643]
          tunnel: [w2642] -> w2631
          frame #0 {
            n1806 = xnode "Read/Write Control"("FPGA VI Reference In"=w2638, "error in"=w2637, "Green Filter Flipper"=TRUE) -> ("FPGA VI Reference Out"=w2635:T19, "error out"=w2634:errorcluster)
          }
          frame #1 {
            n1807 = Wait (ms)(milliseconds to wait=u32 100) -> ()  [unwired: 1 out]
          }
          frame #2 {
            n1808 = xnode "Read/Write Control"("FPGA VI Reference In"=w2644, "error in"=w2643, "Green Filter Flipper"=FALSE) -> ("error out"=w2642:errorcluster)  [unwired: 1 out]
          }
        }
      }
      event "Pump 1 contents", "Pump 3 contents": Value Change {
        n1809 = event-data() -> ()  [unwired: 7 out]
        n1810 = local read "Pump 1 contents"() -> (→"Pump 1 cont disp":string)
        n1811 = local read "Pump 3 contents"() -> (→"Pump 3 cont disp":string)
      }
      event "Reset Trap Pos. FB": Value Change {
        n1812 = event-data() -> ()  [unwired: 7 out]
        n1813 = xnode "Read/Write Control"("FPGA VI Reference In"=w2650, "error in"=w2649, "Trap Pos. FB Reset"="Reset Trap Pos. FB") -> ()  [unwired: 2 out]
      }
      event "Rem fb disp offset": Value Change {
        n1814 = event-data() -> ()  [unwired: 7 out]
        n1815 = local write "Rem fb disp offset"(FALSE ("Rem fb disp offset")) -> ()
        n1816 = local read "Mean T1 Position (nm)"() -> (w2652:dbl)
        n1817 = local read "FB Trap Pos Offset"() -> (w2653:dbl)
        n1818 = Subtract(x=w2653, y=w2652) -> (x-y=w2651:dbl)
        n1819 = local write "FB Trap Pos Offset"(w2651) -> ()
      }
      event "Threshold (nm)": Value Change {
        n1820 = event-data() -> ()  [unwired: 7 out]
        n1821 = flat-sequence {
          tunnel: w2657 -> [w2665]
          tunnel: w2656 -> [w2664]
          tunnel: [w2658] -> w2655
          tunnel: w2655 -> [w2671]
          frame #0 {
            n1822 = xnode "Read/Write Control"("FPGA VI Reference In"=w2665, "error in"=w2664) -> ("FPGA VI Reference Out"=w2661:T19, "error out"=w2660:errorcluster, "FPGA TTrig Thresh"=w2662:i64)
            n1823 = local read "Threshold stored (nm)"() -> (w2670:dbl)
            n1824 = local read "Threshold (nm)"() -> (w2658:dbl)
            n1825 = local read "AOM X Cal (nm/MHz)"() -> (w2668:dbl)
            n1826 = Subtract(x=w2658, y=w2670) -> (x-y=w2669:dbl)
            n1827 = Divide(x=w2669, y=w2668) -> (x/y=w2666:dbl)
            n1828 = call "IR AOM freq to word.vi"("Frequency In (MHz)"=w2666) -> ("Frequency Word Out (double)"=w2667:dbl)
            n1829 = To Quad Integer(1:w2667) -> (0:w2663:i64)
            n1830 = Add(x=w2662, y=w2663) -> (x+y=w2659:i64)
            n1831 = xnode "Read/Write Control"("FPGA VI Reference In"=w2661, "error in"=w2660, "FPGA TTrig Thresh"=w2659) -> ()  [unwired: 2 out]
          }
          frame #1 {
            "Threshold stored (nm)" <- w2671
          }
        }
      }
      event "FB Trig Integrate": Value Change {
        n1832 = event-data() -> ()  [unwired: 7 out]
        n1833 = local read "FB Trig Integrate"() -> (w2673:u32)
        n1834 = xnode "Read/Write Control"("FPGA VI Reference In"=w2675, "error in"=w2674, "FB Trig Integrate"=w2673) -> ("error out"=w2672:errorcluster)  [unwired: 1 out]
      }
      event "11": Value Change {
        n1835 = event-data() -> ()  [unwired: 7 out]
        n1836 = local read "11"() -> (w2676:bool)
        n1837 = case shown="True" w2676 {
          frame False {
          }
          frame True {
            n1838 = local read "Messages"() -> (w2678:string)
            n1839 = call "Update messages.vi"("Message to add"="You kicked it up to 11!", "Old message string"=w2678) -> ("New message string"=w2679:string)
            n1840 = call <vilib>:"Beep.vi"() -> ()  [unwired: 12 in]
            n1841 = local write "Messages"(w2679) -> ()
          }
        }
      }
      event "Trap Pos. FB ON": Value Change {
        n1842 = event-data() -> ()  [unwired: 7 out]
        n1843 = xnode "Read/Write Control"("FPGA VI Reference In"=w2682, "error in"=w2681, "Force feedback"="Trap Pos. FB ON") -> ()  [unwired: 2 out]
      }
      event "Remove Action Offset": Value Change {
        n1844 = event-data() -> ()  [unwired: 7 out]
        n1845 = local write "Remove Action Offset"(FALSE ("Remove Action Offset")) -> ()
        n1846 = local read "Trap Pos. FB Mult Factor"() -> (w2687:i64)
        n1847 = local read "Trap Pos FB Action"() -> (w2685:i64)
        n1848 = local read "Trap Pos. FB Offset Factor"() -> (w2683:i64)
        n1849 = Multiply(x=w2687, y=w2685) -> (x*y=w2686:i64)
        n1850 = Add(x=w2686, y=w2683) -> (x+y=w2684:i64)
        n1851 = local write "Trap Pos. FB Offset Factor"(w2684) -> ()
        n1852 = xnode "Read/Write Control"("FPGA VI Reference In"=w2690, "error in"=w2689, "Trap Pos. FB Offset Factor"=w2684) -> ()  [unwired: 2 out]
      }
      event "Remove Unwinding Offset": Value Change {
        n1853 = event-data() -> ()  [unwired: 7 out]
        n1854 = local write "Remove Unwinding Offset"(FALSE ("Remove Action Offset")) -> ()
        n1855 = local read "Trap Pos. FB Mult Factor"() -> (w2702:i64)
        n1856 = local read "Trap Pos FB Action"() -> (w2700:i64)
        n1857 = local read "Trap Pos. FB Offset Factor"() -> (w2699:i64)
        n1858 = Multiply(x=w2702, y=w2700) -> (x*y=w2701:i64)
        n1859 = local read "Trap Pos. FB Mult Factor"() -> (w2698:i64)
        n1860 = Add(x=w2701, y=w2699) -> (x+y=w2692:i64)
        n1861 = Multiply(x=32768, y="factor") -> (x*y=w2695:dbl)
        n1862 = Multiply(x=w2695, y=w2698) -> (x*y=w2697:dbl)
        n1863 = Subtract(x=w2692, y=w2697) -> (x-y=w2696:dbl)
        n1864 = To Quad Integer(1:w2696) -> (0:w2691:i64)
        n1865 = xnode "Read/Write Control"("FPGA VI Reference In"=w2705, "error in"=w2704, "Trap Pos. FB Offset Factor"=w2691) -> ()  [unwired: 2 out]
        n1866 = local write "Trap Pos. FB Offset Factor"(w2691) -> ()
      }
      event "Trap Pos. FB Range", "Trap Pos. FB Gains", "Trap Pos. FB Mult Factor", "Trap Pos. FB Offset Factor", "Trap Pos FB Negate Action", "Trap Pos FB Monitor\nT1 or T2", "Differential FB?", "Negate Diff?": Value Change {
        n1867 = event-data() -> ()  [unwired: 7 out]
        n1868 = local read "Negate Diff?"() -> (w2706:bool)
        n1869 = xnode "Read/Write Control"("FPGA VI Reference In"=w2716, "error in"=w2715, "Trap Pos. FB Range"="Trap Pos. FB Range", "Trap Pos. FB Gains"="Trap Pos. FB Gains", "Trap Pos. FB Mult Factor"="Trap Pos. FB Mult Factor", "Trap Pos. FB Offset Factor"="Trap Pos. FB Offset Factor", "Trap Pos FB Negate Action"="Trap Pos FB Negate Action", "Trap Pos FB Monitor T1 or T2"="Trap Pos FB Monitor\nT1 or T2", "AI1 X Scale"="Trap Pos. AI1 X Pre-scale", "Negate Diff?"=w2706, "Diff FB Measurement?"="Differential FB?") -> ()  [unwired: 2 out]
      }
      event "Trap Pos FB SP", "Trap Pos FB SP 2", "Use SP 2": Value Change {
        n1870 = event-data() -> ()  [unwired: 7 out]
        n1871 = Select(t="Trap Pos FB SP 2", s="Use SP 2", f="Trap Pos FB SP") -> (s? t:f=w2717:fxp<+/-,16,1>)
        n1872 = xnode "Read/Write Control"("FPGA VI Reference In"=w2722, "error in"=w2721, "Trap Pos. FB SP"=w2717) -> ()  [unwired: 2 out]
      }
      event "Offset SP2 from SP1": Value Change {
        n1873 = event-data() -> ()  [unwired: 7 out]
        n1874 = local read "Trap Pos FB SP"() -> (w2725:fxp<+/-,16,1>)
        n1875 = Add(x=w2725, y="SP2 Offset") -> (x+y=w2723:fxp<+/-,16,1>)
